vi "Read Element of Views.vi"(8 "error in (no error)":errorcluster, 10 "Index":i32, 11 "IViewManager In":refnum<class "IViewManager.lvclass">) -> (0 "error out":errorcluster, 2 "View Ref":refnum<class "Message Enqueuer.lvclass">, 3 "IViewManager Out":refnum<class "IViewManager.lvclass">)   [LabVIEW 2015, in "IViewManager.lvlib" / "IViewManager.lvclass"]
doc: "<License>\nCopyright © 2017 Composed Systems, LLC | All rights reserved\nwww.composed.io\n\nAuthor: Ethan Stern <ethan.stern@composed.io>\n\nThis software is provided \"AS IS\" WITHOUT WARRANTIES, either express or implied, AND IS FOR EDUCATIONAL PURPOSES ONLY.\n</License>"
uses:
  IViewManager.lvclass
  <vilib>/ActorFramework/Message Enqueuer/Message Enqueuer.lvclass
  IViewManager.lvclass/IViewManager.ctl
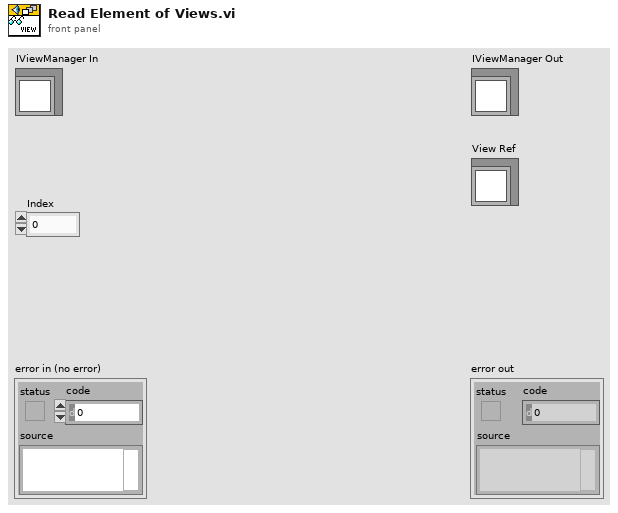
[diagram p1: front panel]
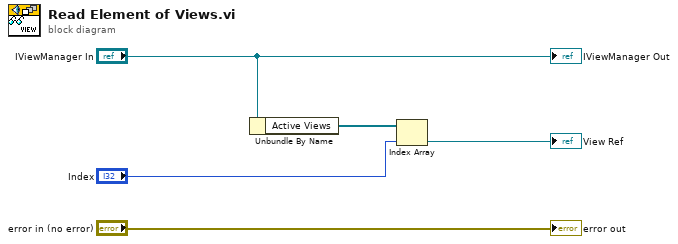
[diagram p0: block diagram]
diagram:
  n1 = Unbundle By Name("IViewManager In") -> ("Active Views"=w1:refnum<class "Message Enqueuer.lvclass">[])
  n2 = Index Array(array=w1, index="Index") -> (element=→"View Ref":refnum<class "Message Enqueuer.lvclass">)
  "error out" <- "error in (no error)"
  "IViewManager Out" <- "IViewManager In"
